vi "FlatToRichgrpcservice_AkipRequest.vi"(5 "OutputClusterType":T1, 11 "InputCluster":T2) -> (3 "OutputCluster":T1)   [LabVIEW 2023, in "Proto_client.lvlib"]
uses:
  grpcservice_AkipRequest_Flat.ctl
  grpcservice_AkipRequest.ctl
  Proto_client.lvlib
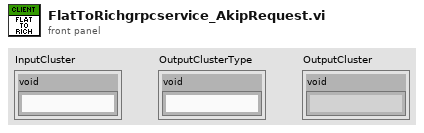
[diagram p1: front panel]
types:
  T1 = typedef "Proto_client.lvlib/grpcservice_AkipRequest.ctl" = cluster{"void":string}
  T2 = typedef "Proto_client.lvlib/grpcservice_AkipRequest_Flat.ctl" = cluster{"void":string}
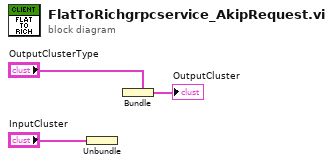
[diagram p0: block diagram]
diagram:
  n1 = Unbundle "Unbundle"("InputCluster") -> ()  [unwired: 1 out]
  n2 = Bundle "Bundle"(cluster="OutputClusterType") -> (→"OutputCluster":T1)  [unwired: 1 in]
